vi "报表存储.vi"() -> ()   [LabVIEW 2013]
uses:
  <vilib>/printing/EasyPrintingControls.llb/contents.ctl
  <vilib>/Utility/NIReport.llb/NI_ReportGenerationCore.lvlib
  <vilib>/printing/EasyPrintingControls.llb/report_type.ctl
  <vilib>/printing/EasyPrinting.llb/Easy Print VI Panel or Documentation (path).vi
  <vilib>/Utility/NIReport.llb/NI_report.lvclass
panel:
  out "error out 5":errorcluster caption="错误输出"
  out "推拉力数组":dbl[](array[numeric])
  out "位移数据":dbl[](array[numeric])
  out "间隙数组":dbl[](array[numeric])
  out "扭矩数组":dbl[](array[numeric])
  in  "产品ID":string="201209190001"
  in  "工步号":u32
types:
  T1 = typedef "NI_ReportGenerationCore.lvlib/report_type.ctl" = u16
  T2 = typedef "NI_ReportGenerationCore.lvlib/contents.ctl" = u16
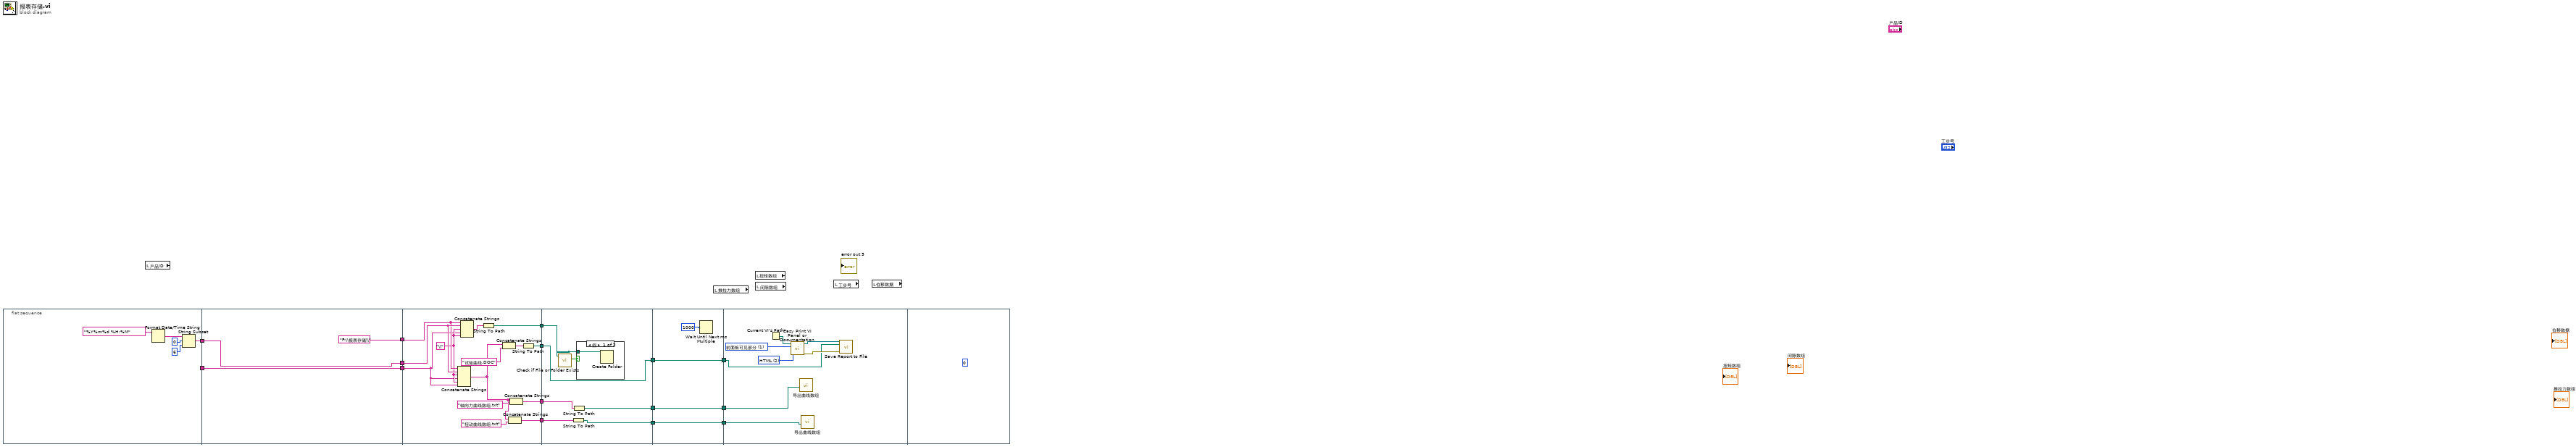
[diagram p0: block diagram]
diagram:
  n1 = flat-sequence {
    tunnel: [w21] -> w19
    tunnel: [w20] -> w18
    tunnel: w19 -> [w28]
    tunnel: w18 -> [w27]
    tunnel: [w28] -> w17
    tunnel: [w27] -> w16
    tunnel: ["F:\\报表存储\\" ("字符串")] -> w15
    tunnel: w17 -> [w41]
    tunnel: w16 -> [w34]
    tunnel: w15 -> [w40]
    tunnel: [w39] -> w14
    tunnel: [w36] -> w13
    tunnel: [w30] -> w12
    tunnel: [w29] -> w11
    tunnel: w14 -> [w47]
    tunnel: [w48] -> w10
    tunnel: w13 -> [w48]
    tunnel: w12 -> [w46]
    tunnel: w11 -> [w45]
    tunnel: [w44] -> w9
    tunnel: [w43] -> w8
    tunnel: [w53] -> w7
    tunnel: w10 -> [w53]
    tunnel: w9 -> [w52]
    tunnel: [w52] -> w6
    tunnel: [w51] -> w5
    tunnel: w8 -> [w51]
    tunnel: w7 -> [w61]
    tunnel: w6 -> [w58]
    tunnel: w5 -> [w55]
    frame #0 {
      n2 = Format Date/Time String(time format string (%c)="%Y%m%d %H:%M" ("时间格式字符串(%c)")) -> (date/time string=w22:string)  [unwired: 2 in]
      n3 = String Subset(string=w22, offset (0)=0 ("偏移量(0)"), length (rest)=6 ("长度（剩余）")) -> (substring=w21:string)
    }
    frame #1 {
    }
    frame #2 {
      w35 = "\\" ("字符串")
      n4 = Concatenate Strings(w40, w41, w35, w34, w35, w34) -> (w32:string)
      n5 = Concatenate Strings(w40, w41, w35, w34, w35) -> (w42:string)
      n6 = String To Path(string=w42) -> (path=w39:path)
      n7 = Concatenate Strings(w32, "试验曲线.DOC" ("字符串")) -> (w37:string)
      n8 = Concatenate Strings(w32, "扭动曲线数组.txt" ("字符串")) -> (w29:string)
      n9 = Concatenate Strings(w32, "轴向力曲线数组.txt" ("字符串")) -> (w30:string)
      n10 = String To Path(string=w37) -> (path=w36:path)
    }
    frame #3 {
      n11 = call <vilib>:"Check if File or Folder Exists.vi"("path"=w47) -> ("file or folder exists?"=w49:bool)  [unwired: 8 in, 2 out]
      n12 = String To Path(string=w45) -> (path=w43:path)
      n13 = String To Path(string=w46) -> (path=w44:path)
      n14 = case shown="假" w49 {
        tunnel: w47 -> [w50 _]
        frame False {
          n15 = Create Folder(path (use dialog)=w50) -> ()  [unwired: 2 in, 3 out]
        }
        frame True {
        }
      }
    }
    frame #4 {
      n16 = Wait Until Next ms Multiple(millisecond multiple=u32 1000 ("毫秒倍数")) -> ()  [unwired: 1 out]
    }
    frame #5 {
      w64 = T1 2 items=["快速打印", "标准报表", "HTML", "双字节", "Excel"] ("report type (Quick Print)")
      w63 = T2 1 items=["完整前面板", "前面板可见部分", "图标、说明、前面板和程序框图", "说明信息: 使用前面板", "说明信息: 作为子VI使用", "说明信息: 完整", "说明信息: 自定义"] ("contents (complete front panel)")
      n17 = Current VI's Path() -> (path=w62:path)
      n18 = call-poly <vilib>:"Easy Print VI Panel or Documentation.vi"("report type (Quick Print)"=w64, "contents (complete front panel)"=w63, "VI path"=w62) -> ("error out"=w66:errorcluster, "report out"=w65:refnum<class "NI_report.lvclass">)  [unwired: 1 in, 6 out]
      n19 = call "导出曲线数组.vi"("file path (dialog if empty)"=w58) -> ("数组 2"=w59:dbl[], "数组"=w60:dbl[])  [unwired: 9 in]
      n20 = call "导出曲线数组.vi"("file path (dialog if empty)"=w55) -> ("数组 2"=w56:dbl[], "数组"=w57:dbl[])  [unwired: 9 in]
      n21 = call-dynamic "Save Report to File.vi"("report in"=w65, "report file path"=w61, "error in (no error)"=w66) -> ("error out"=w67:errorcluster)  [unwired: 2 in, 10 out]
    }
    frame #6 {
      (unwired) u32 0 ("工步号")
    }
  }
  n22 = local read "产品ID"() -> ()  [unwired: 1 out]
  n23 = local read "推拉力数组"() -> (w1:dbl[])
  n24 = local read "扭矩数组"() -> (w2:dbl[])
  n25 = local read "间隙数组"() -> (w3:dbl[])
  n26 = local read "工步号"() -> (w4:u32)
  n27 = local read "位移数据"() -> ()  [unwired: 1 out]
